vi "SpreadsheetStorageKundts.vi"(0 "input cluster":cluster{"Freq":i16[], "Gain":dbl[]}) -> ()   [LabVIEW 2014]
uses:
  <vilib>/Utility/file.llb/Write To Spreadsheet File (DBL).vi
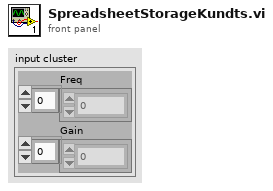
[diagram p1: front panel]
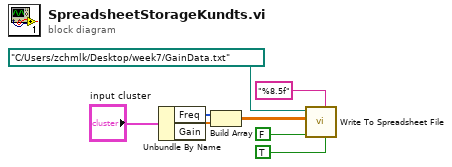
[diagram p0: block diagram]
diagram:
  n1 = Unbundle By Name("input cluster") -> ("Freq"=w3:i16[], "Gain"=w4:dbl[])
  n2 = Build Array(w3, w4) -> (w7:dbl[][])
  n3 = call-poly <vilib>:"Write To Spreadsheet File.vi"("transpose? (no:F)"=TRUE, "format (%.3f)"="%8.5f", "append to file? (new file:F)"=FALSE, "2D data"=w7, "file path (dialog if empty)"=path "C:/Users/zchmlk/Desktop/week7/GainData.txt") -> ()  [unwired: 3 in, 1 out]
